vi "Diode-Test.vi"() -> ()   [LabVIEW 2020]
uses:
  Diode-SCPI-Driver/Diode-Keyword.ctl
panel:
  in  "Diode Keyword":T1={"Keyword"="*IDN", "Gettable"=TRUE, "Settable"=FALSE, "Is Array"=FALSE, "Data Type"="string", "Description"="Identify the instrument."}
  out "Response":string
  in  "IP Address of Device":string="192.168.203.151"
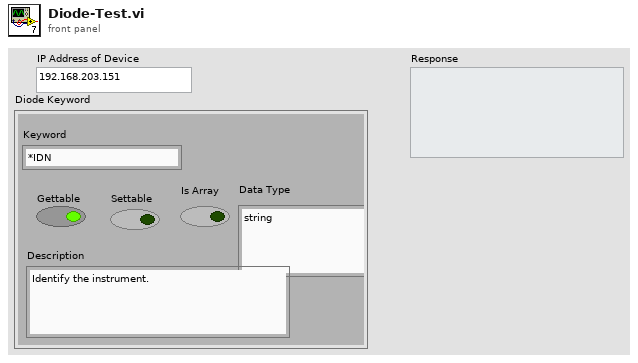
[diagram p1: front panel]
types:
  T1 = typedef "Diode-Keyword.ctl" = cluster{"Keyword":string, "Gettable":bool, "Settable":bool, "Is Array":bool, "Data Type":string, "Description":string}
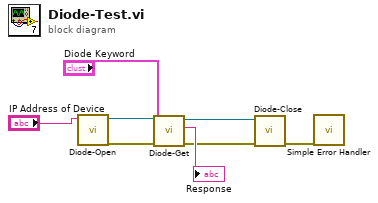
[diagram p0: block diagram]
diagram:
  n1 = call "Diode-Open.vi"("IP Address of Diode"="IP Address of Device") -> ("error out"=w1:errorcluster, "connection ID"=w4:refnum<k5>)  [unwired: 9 in]
  n2 = call "Diode-Get.vi"("error in (no error)"=w1, "Diode Keyword (leave off question mark)"="Diode Keyword", "connection ID"=w4) -> ("error out"=w2:errorcluster, "Response"=→"Response":string, "connection ID out"=w3:refnum<k5>)  [unwired: 5 in, 1 out]
  n3 = call "Diode-Close.vi"("error in (no error)"=w2, "connection ID"=w3) -> ("error out"=w7:errorcluster)  [unwired: 9 in]
  n4 = call <vilib>:"Simple Error Handler.vi"("error in (no error)"=w7) -> ()  [unwired: 4 in, 5 out]
